vi "Read channels.vi"(8 "error in (no error)":errorcluster, 11 "DSFConfiguration in":refnum<class "DSFConfiguration.lvclass">) -> (0 "error out":errorcluster, 2 "channels":cluster{"id":string, "values":T1}[](array[cluster]), 3 "DSFConfiguration out":refnum<class "DSFConfiguration.lvclass">)   [LabVIEW 2017, in "DSFConfiguration.lvclass"]
uses:
  DSFConfiguration.lvclass
  Controls/dsf configuration file/1.0.0/dsf channel.ctl
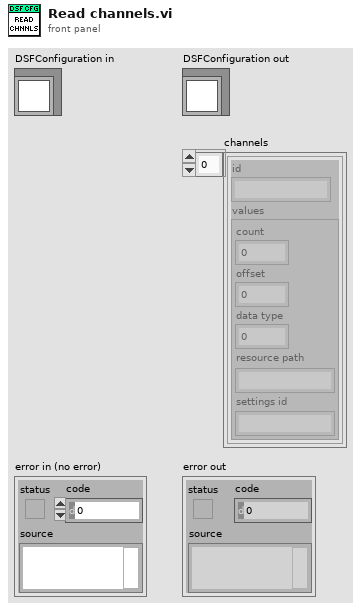
[diagram p1: front panel]
types:
  T1 = typedef "dsf configuration file v1.0.0.lvlib/dsf channel.ctl" = cluster{"count":i32, "offset":i32, "data type":dbl, "resource path":string, "settings id":string}
  T2 = typedef "dsf configuration file v1.0.0.lvlib/dsf channel.ctl" = cluster{"id":string, "values":cluster{"count":i32, "offset":i32, "data type":i32, "resource path":string, "settings id":string}}
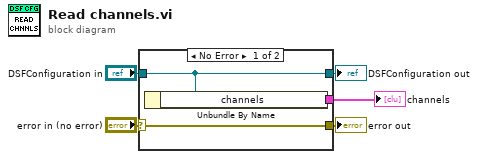
[diagram p0: block diagram]
diagram:
  n1 = case shown="No Error" "error in (no error)" {
    selector: "error in (no error)" -> [w8 w9]
    tunnel: [w8 w9] -> w4
    tunnel: [w7 w10] -> w2
    tunnel: "DSFConfiguration in" -> [w7 w10]
    tunnel: [w6 _] -> w1
    frame No Error {
      n2 = Unbundle By Name(w7) -> ("channels"=w6:T2[])
    }
    frame Error {
    }
  }
  "error out" <- w4
  "DSFConfiguration out" <- w2
  "channels" <- w1
